vi "get update log.vi"(8 "error in (no error)":errorcluster caption="错误输入（无错误）", 11 "服务器信息":T1={"host"="27.154.58.30", "port"=8020, "user"="std", "password"="std23506", "远端地址"="/微站/室外总磷总氮高压过滤无主板新电路板/一体化微型水质监测站.exe"}) -> (0 "error out":errorcluster caption="错误输出", 1 "部分更新日志":string, 2 "remote File Version":string, 3 "更新日志":string, 5 "MD5":string)   [LabVIEW 2016, in "数据传输系统.lvlib" / "update.lvlib"]
uses:
  update.lvlib
  <vilib>/regexp/Match Regular Expression.xnode
  <vilib>/httpClient/LabVIEWHTTPClient.lvlib
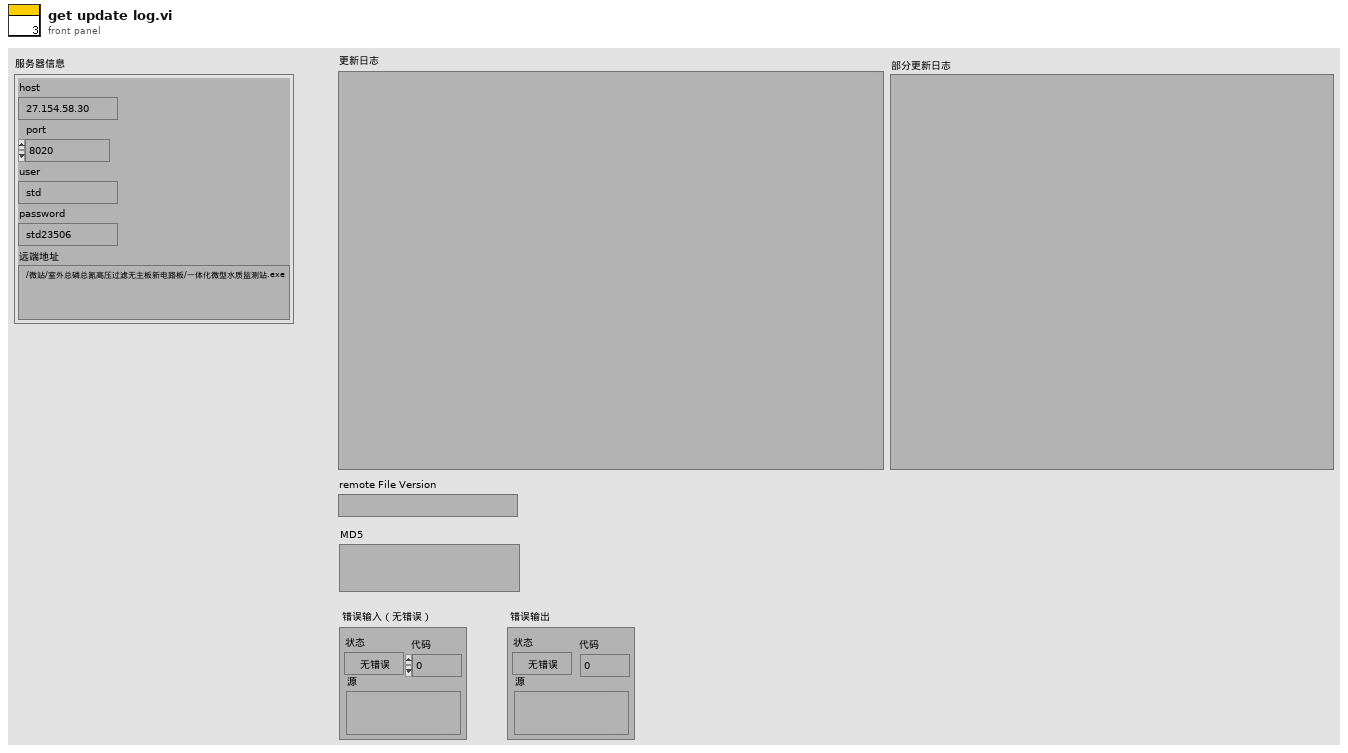
[diagram p1: front panel]
types:
  T1 = cluster{"host":string, "port":u16, "user":string, "password":string, "远端地址":string}
  T2 = typedef "LabVIEWHTTPClient.lvlib/ClientHandle.ctl" = refnum<k1>
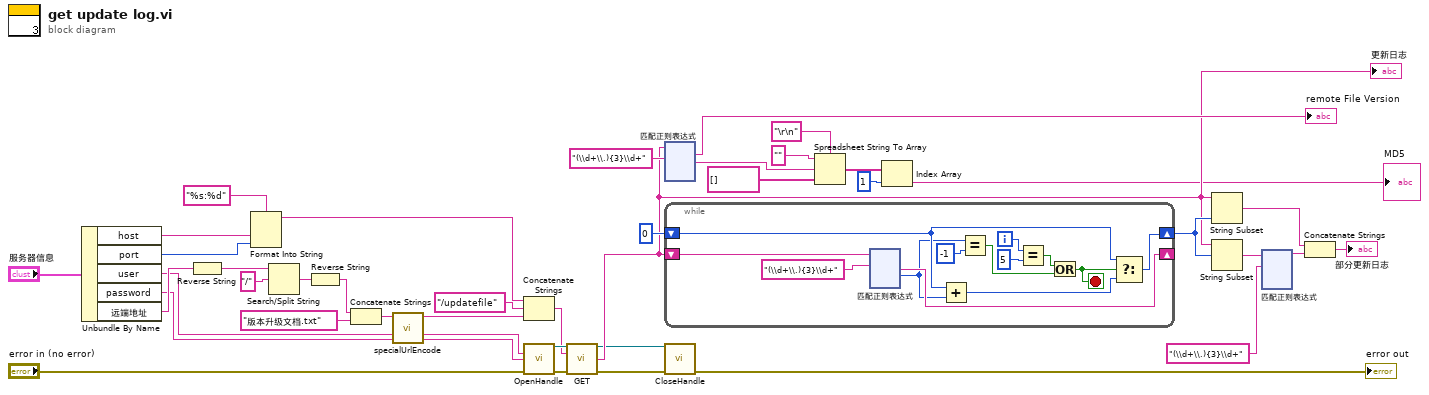
[diagram p0: block diagram]
diagram:
  n1 = Unbundle By Name("服务器信息") -> ("host"=w16:string, "port"=w15:u16, "user"=w19:string, "password"=w20:string, "远端地址"=w26:string)
  n2 = Reverse String(1:w26) -> (0:w37:string)
  n3 = Format Into String(format string="%s:%d" ("格式字符串"), w16, w15) -> (resulting string=w14:string)  [unwired: 2 in, 1 out]
  n4 = Search/Split String(string=w37, search string/char (-)="/" ("搜索字符串/字符(-)")) -> (match + rest of string=w35:string)  [unwired: 1 in, 2 out]
  n5 = Reverse String(1:w35) -> (0:w34:string)
  n6 = Concatenate Strings(w34, "版本升级文档.txt" ("字符串")) -> (w18:string)
  n7 = call "specialUrlEncode.vi"("str"=w18) -> ("UrlEncode"=w17:string)  [unwired: 10 in]
  n8 = Concatenate Strings(w14, "/updatefile", w17) -> (w12:string)
  n9 = call <vilib>:"OpenHandle.vi"("username"=w19, "password"=w20, "error in (no error)"="error in (no error)") -> ("client handle out"=w25:T2, "error out"=w24:errorcluster)  [unwired: 11 in]
  n10 = call <vilib>:"GET.vi"("client handle"=w25, "url"=w12, "error in (no error)"=w24) -> ("client handle out"=w8:T2, "body"=w23:string, "error out"=w10:errorcluster)  [unwired: 9 in, 1 out]
  "更新日志" <- w23
  n11 = xnode "匹配正则表达式"("输入字符串"=w23, "正则表达式"="(\\d+\\.){3}\\d+") -> ("所有匹配"=→"remote File Version":string, "匹配之后"=w5:string)  [unwired: 4 in, 3 out]
  n12 = while {
    shift-right: [w50] -> _
    shift-left: w23 -> [w52]
    shift-right: [w51] -> w30
    shift-left: 0 ("匹配后偏移量") -> [w48]
    i -> [w47]
    stop <- w46 stop-if-true
    n13 = xnode "匹配正则表达式"("输入字符串"=w52, "正则表达式"="(\\d+\\.){3}\\d+") -> ("匹配之后"=w50:string, "匹配后偏移量"=w41:i32)  [unwired: 4 in, 3 out]
    n14 = Add(x=w48, y=w41) -> (x+y=w49:i32)
    n15 = Equal?(x=w41, y=-1) -> (x = y?=w43:bool)
    n16 = Equal?(x=w47, y=5) -> (x = y?=w45:bool)
    n17 = Or(x=w45, y=w43) -> (x .or. y?=w46:bool)
    n18 = Select(t=w48, s=w46, f=w49) -> (s? t:f=w51:i32)
  }
  n19 = call <vilib>:"CloseHandle.vi"("client handle"=w8, "error in (no error)"=w10) -> ("error out"=→"error out":errorcluster)  [unwired: 13 in]
  n20 = Spreadsheet String To Array(delimiter (Tab)="\r\n" ("分隔符(Tab)"), format string="", spreadsheet string=w5, array type (2D Dbl)=string[] []) -> (array=w3:string[])
  n21 = Index Array(array=w3, index=1 ("索引")) -> (element=→"MD5":string)
  n22 = String Subset(string=w23, length (rest)=w30) -> (substring=w28:string)  [unwired: 1 in]
  n23 = String Subset(string=w23, offset (0)=w30) -> (substring=w31:string)  [unwired: 1 in]
  n24 = xnode "匹配正则表达式"("输入字符串"=w31, "正则表达式"="(\\d+\\.){3}\\d+") -> ("匹配之前"=w29:string)  [unwired: 4 in, 4 out]
  n25 = Concatenate Strings(w28, w29) -> (→"部分更新日志":string)
